vi "velocity profile.vi"(6 "Konstant":dbl=2.0 format="%#_13g", 8 "Max Accel":dbl, 9 "Max Vel":dbl, 10 "Curvatures":dbl[](array[numeric]), 11 "Distances":dbl[](array[numeric])) -> (2 "Max Velocities":dbl[](array[numeric]), 3 "Target Velocities":dbl[](array[numeric]))   [LabVIEW 2018]
panel:
  out "Target Velocities":dbl[](graph)
  out "Max Velocities":dbl[](graph)
  out "element":dbl
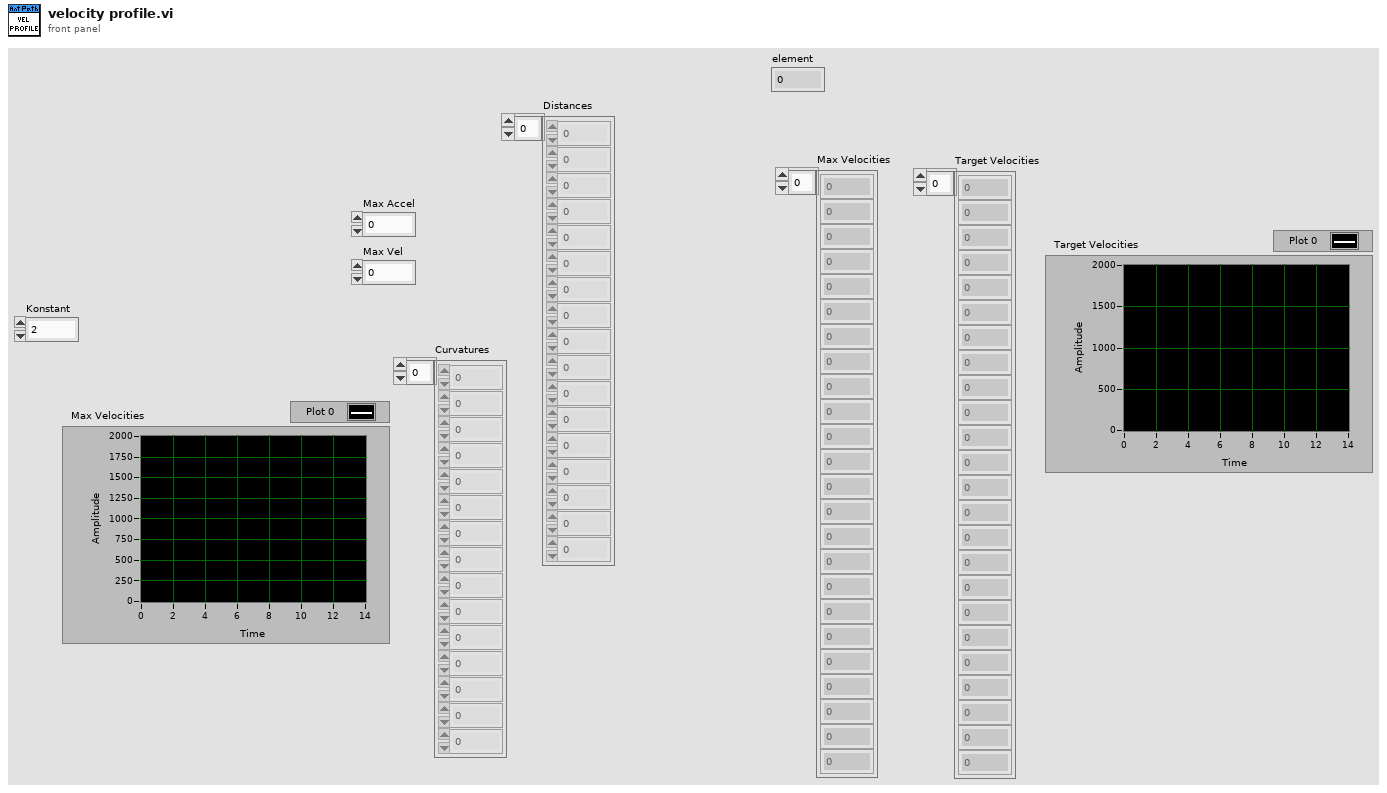
[diagram p1: front panel]
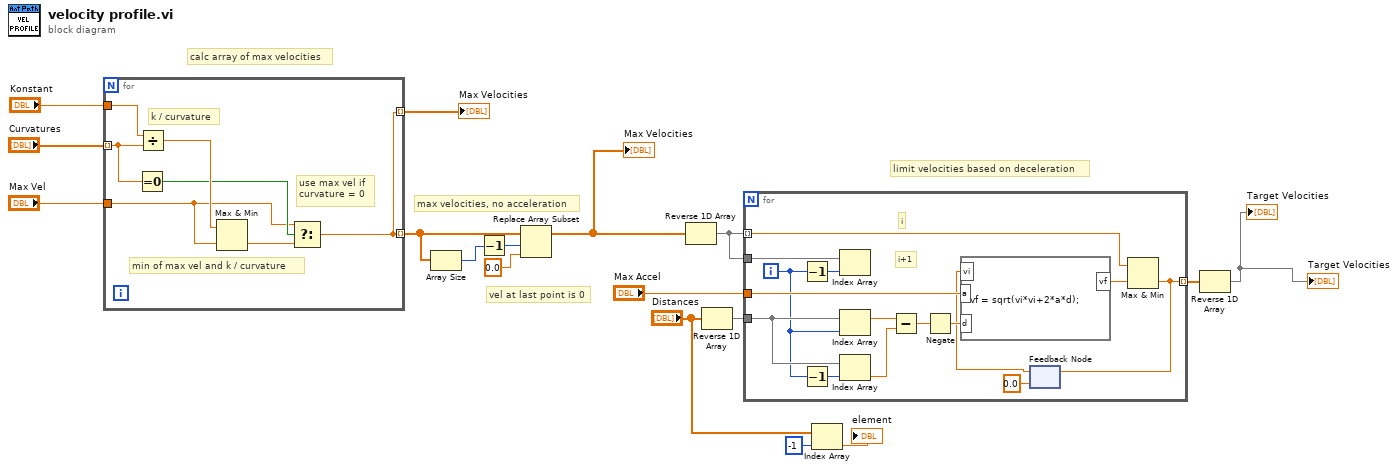
[diagram p0: block diagram]
diagram:
  # "limit velocities based on deceleration"
  # "calc array of max velocities"
  # "vel at last point is 0"
  # "max velocities, no acceleration"
  n1 = for {
    tunnel: "Curvatures" -> [w22] mode=indexing
    tunnel: "Max Vel" -> [w19]
    tunnel: [w18] -> w11 mode=indexing
    tunnel: "Konstant" -> [w20]
    tunnel: [w18] -> w2 mode=indexing
    # "min of max vel and k / curvature"
    # "use max vel if \ncurvature = 0"
    # "k / curvature"
    n2 = Equal To 0?(x=w22) -> (x = 0?=w23:bool)
    n3 = Divide(x=w20, y=w22) -> (x/y=w24:dbl)
    n4 = Max & Min(x=w24, y=w19) -> (min(x,y)=w21:dbl)  [unwired: 1 out]
    n5 = Select(t=w19, s=w23, f=w21) -> (s? t:f=w18:dbl)
  }
  "Max Velocities" <- w2
  n6 = Array Size(array=w11) -> (size(s)=w8:i32)
  n7 = Decrement(x=w8) -> (x-1=w10:i32)
  n8 = Replace Array Subset(array=w11, new element=0.0 ("new element/subarray"), index=w10) -> (w3:dbl[])
  "Max Velocities" <- w3
  n9 = Reverse 1D Array(array=w3) -> (reversed array=w13:dbl[])
  n10 = Reverse 1D Array(array="Distances") -> (reversed array=w14:dbl[])
  n11 = for {
    tunnel: w14 -> [w29]
    tunnel: "Max Accel" -> [w37]
    tunnel: w13 -> [w30] mode=indexing
    tunnel: w13 -> [w36]
    tunnel: [w25] -> w9 mode=indexing
    i -> [w28]
    # "i"
    # "i+1"
    n12 = Decrement(x=w28) -> (x-1=w33:i32)
    n13 = Decrement(x=w28) -> (x-1=w31:i32)
    n14 = Index Array(array=w36, index=w33) -> ()  [unwired: 1 out]
    n15 = Index Array(array=w29, index=w28) -> (element=w35:dbl)
    n16 = Index Array(array=w29, index=w31) -> (element=w32:dbl)
    n17 = Subtract(x=w35, y=w32) -> (x-y=w39:dbl)
    n18 = Negate(x=w39) -> (-x=w34:dbl)
    n19 = feedback #1(0.0) -> (w26:dbl)
    n20 = formula code="vf = sqrt(vi*vi+2*a*d);"("vi"=w26, "a"=w37, "d"=w34) -> ("vf"=w38:dbl)
    n21 = Max & Min(x=w30, y=w38) -> (min(x,y)=w25:dbl)  [unwired: 1 out]
    n22 = feedback-in #1(w25) -> ()
  }
  n23 = Index Array(array="Distances", index=-1) -> (element=→"element":dbl)
  n24 = Reverse 1D Array(array=w9) -> (reversed array=→"Target Velocities" →"Target Velocities":dbl[])
